vi "Message to Display String.vi"(1 "Message":T1) -> (0 "message string":string)   [LabVIEW 2019, in "RemoteControl.lvclass"]
uses:
  RemoteControl.lvclass
  Typedefs/Message--Cluster.ctl
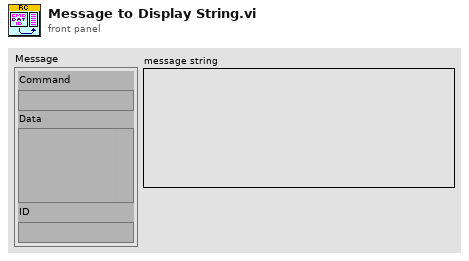
[diagram p1: front panel]
types:
  T1 = typedef "RemoteControl.lvclass/Message--Cluster.ctl" = cluster{"Command":string, "Data":variant, "ID":string}
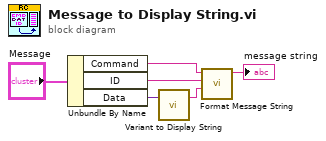
[diagram p0: block diagram]
diagram:
  n1 = Unbundle By Name("Message") -> ("Command"=w4:string, "ID"=w3:string, "Data"=w5:variant)
  n2 = call "Variant to Display String.vi"("Variant"=w5) -> ("xml string"=w2:string)  [unwired: 2 in]
  n3 = call "Format Message String.vi"("ID"=w2, "Data"=w3, "Command"=w4) -> ("Message"=→"message string":string)  [unwired: 8 in]
